vi "Array Sizer.vi"(2 "maxV":dbl=20.0 step=5.0, 3 "Angular Accelerations":T1 {"Angular \nAccelerations" step=5.0}, 4 "Velocities":dbl[](array[numeric]) step=5.0, 5 "Points out":cluster{"x":dbl, "y":dbl, "th":dbl}[](array[cluster])) -> (0 "Velocities out":dbl[](array[numeric]) step=5.0, 1 "output cluster":T1)   [LabVIEW 2019]
panel:
  # "TURN Acceleration"
  # "1"
  # "1"
  # "2"
  # "2"
  # "3"
  # "3"
  # "4"
  # "4"
  # "5"
  # "5"
  # "6"
  # "6"
  # "7"
  # "7"
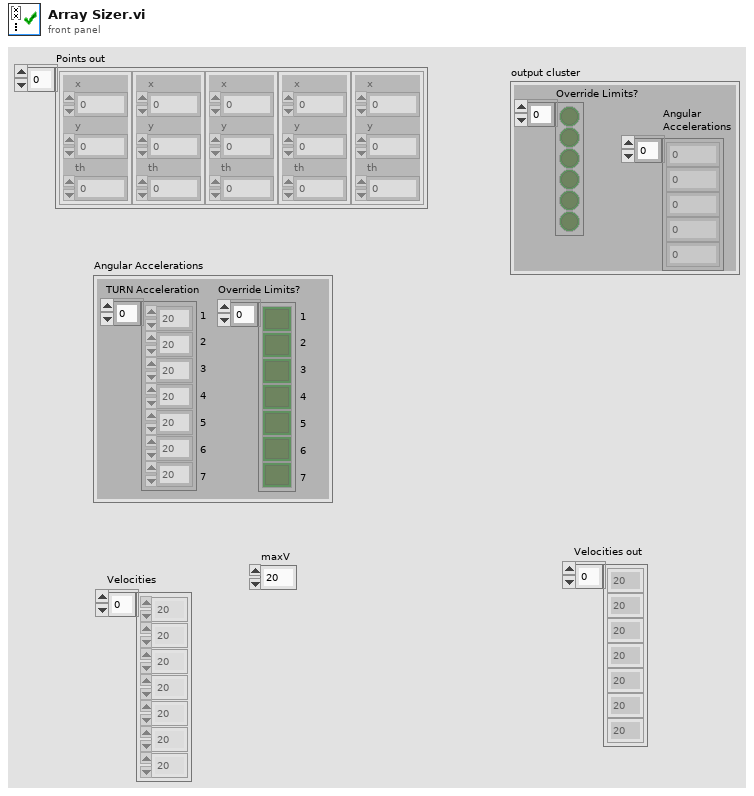
[diagram p1: front panel]
types:
  T1 = cluster{"Angular \nAccelerations":dbl[], "Override Limits?":bool[]}
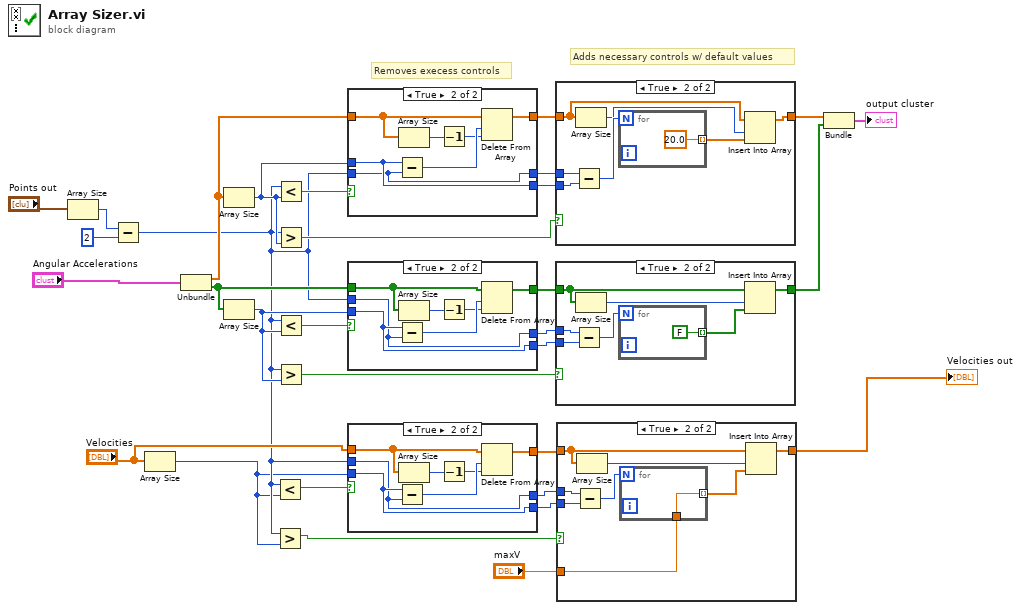
[diagram p0: block diagram]
diagram:
  # "Adds necessary controls w/ default values"
  # "Removes execess controls"
  n1 = Array Size(array="Points out") -> (size(s)=w13:i32)
  n2 = Subtract(x=w13, y=2) -> (x-y=w8:i32)
  n3 = Array Size(array="Velocities") -> (size(s)=w7:i32)
  n4 = Unbundle("Angular Accelerations") -> ("Angular \nAccelerations"=w27:dbl[], "Override Limits?"=w20:bool[])
  n5 = Array Size(array=w27) -> (size(s)=w26:i32)
  n6 = Array Size(array=w20) -> (size(s)=w19:i32)
  n7 = Less?(x=w8, y=w7) -> (x < y?=w10:bool)
  n8 = Greater?(x=w8, y=w7) -> (0:w2:bool)
  n9 = Less?(x=w8, y=w26) -> (x < y?=w30:bool)
  n10 = Greater?(x=w8, y=w26) -> (0:w29:bool)
  n11 = Less?(x=w8, y=w19) -> (x < y?=w14:bool)
  n12 = Greater?(x=w8, y=w19) -> (0:w15:bool)
  n13 = case shown="True" w30 {
    tunnel: [w34 w35] -> w28
    tunnel: w27 -> [w34 w38]
    tunnel: w8 -> [w33 w40]
    tunnel: w26 -> [w32 w41]
    tunnel: [w33 w40] -> w25
    tunnel: [w32 w41] -> w24
    frame False {
    }
    frame True {
      n14 = Subtract(x=w41, y=w40) -> (x-y=w39:i32)
      n15 = Array Size(array=w38) -> (size(s)=w37:i32)
      n16 = Decrement(x=w37) -> (x-1=w36:i32)
      n17 = Delete From Array(array=w38, length=w39, index=w36) -> (array with subset deleted=w35:dbl[])  [unwired: 1 out]
    }
  }
  n18 = case shown="True" w14 {
    tunnel: [w44 w45] -> w21
    tunnel: w20 -> [w44 w48]
    tunnel: w8 -> [w43 w50]
    tunnel: w19 -> [w42 w51]
    tunnel: [w43 w50] -> w22
    tunnel: [w42 w51] -> w23
    frame False {
    }
    frame True {
      n19 = Subtract(x=w51, y=w50) -> (x-y=w49:i32)
      n20 = Array Size(array=w48) -> (size(s)=w47:i32)
      n21 = Decrement(x=w47) -> (x-1=w46:i32)
      n22 = Delete From Array(array=w48, length=w49, index=w46) -> (array with subset deleted=w45:bool[])  [unwired: 1 out]
    }
  }
  n23 = case shown="True" w10 {
    tunnel: [w54 w55] -> w6
    tunnel: "Velocities" -> [w54 w58]
    tunnel: w8 -> [w53 w60]
    tunnel: w7 -> [w52 w61]
    tunnel: [w53 w60] -> w4
    tunnel: [w52 w61] -> w3
    frame False {
    }
    frame True {
      n24 = Subtract(x=w61, y=w60) -> (x-y=w59:i32)
      n25 = Array Size(array=w58) -> (size(s)=w57:i32)
      n26 = Decrement(x=w57) -> (x-1=w56:i32)
      n27 = Delete From Array(array=w58, length=w59, index=w56) -> (array with subset deleted=w55:dbl[])  [unwired: 1 out]
    }
  }
  n28 = case shown="True" w29 {
    tunnel: [w62 w66] -> w18
    tunnel: w28 -> [w62 w65]
    tunnel: w25 -> [_ w69]
    tunnel: w24 -> [_ w68]
    frame False {
    }
    frame True {
      n29 = Subtract(x=w69, y=w68) -> (x-y=w67:i32)
      n30 = Array Size(array=w65) -> (size(s)=w64:i32)
      n31 = for {
        N: w67 -> [_]
        tunnel: [20.0] -> w63 mode=indexing
      }
      n32 = Insert Into Array(array=w65, index=w64, new element=w63) -> (w66:dbl[])
    }
  }
  n33 = case shown="True" w15 {
    tunnel: [w71 w75] -> w17
    tunnel: w21 -> [w71 w74]
    tunnel: w22 -> [_ w78]
    tunnel: w23 -> [_ w77]
    frame False {
    }
    frame True {
      n34 = Subtract(x=w78, y=w77) -> (x-y=w76:i32)
      n35 = Array Size(array=w74) -> (size(s)=w73:i32)
      n36 = for {
        N: w76 -> [_]
        tunnel: [FALSE] -> w72 mode=indexing
      }
      n37 = Insert Into Array(array=w74, index=w73, new element=w72) -> (w75:bool[])
    }
  }
  n38 = case shown="True" w2 {
    tunnel: [w80 w85] -> w5
    tunnel: w6 -> [w80 w84]
    tunnel: w4 -> [_ w88]
    tunnel: w3 -> [_ w87]
    tunnel: "maxV" -> [_ w81]
    frame False {
    }
    frame True {
      n39 = Subtract(x=w88, y=w87) -> (x-y=w86:i32)
      n40 = Array Size(array=w84) -> (size(s)=w83:i32)
      n41 = for {
        N: w86 -> [_]
        tunnel: [w89] -> w82 mode=indexing
        tunnel: w81 -> [w89]
      }
      n42 = Insert Into Array(array=w84, index=w83, new element=w82) -> (w85:dbl[])
    }
  }
  "Velocities out" <- w5
  n43 = Bundle("Angular \nAccelerations"=w18, "Override Limits?"=w17) -> (→"output cluster":T1)  [unwired: 1 in]
